vi "Path Array to Tree.vi"(7 "Path":path, 11 "Tree in":variant) -> (3 "Tree out":variant)   [LabVIEW 2023, in "VIDoc Printer.lvlib" / "VIDoc Printer.lvclass"]
uses:
  VIDoc Printer.lvclass
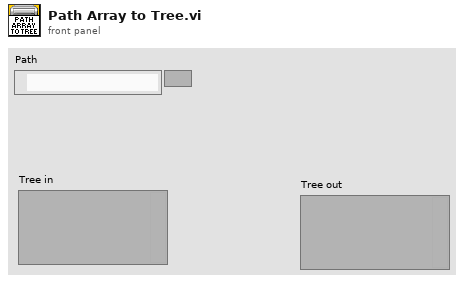
[diagram p1: front panel]
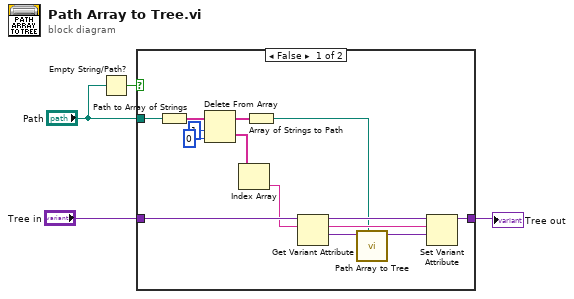
[diagram p0: block diagram]
diagram:
  n1 = Empty String/Path?(string/path="Path") -> (empty?=w2:bool)
  n2 = case shown="False" w2 {
    tunnel: [w16 w18] -> w4
    tunnel: "Tree in" -> [w13 w18]
    tunnel: "Path" -> [w12 _]
    frame False {
      n3 = Path to Array of Strings(0:w12) -> (2:w11:string[])  [unwired: 1 out]
      n4 = Delete From Array(array=w11, length=1, index=0) -> (deleted portion=w8:string[], array with subset deleted=w6:string[])
      n5 = Index Array(array=w8) -> (element=w7:string)  [unwired: 1 in]
      n6 = Array of Strings to Path(0:w6) -> (2:w5:path)  [unwired: 1 in]
      n7 = Get Variant Attribute(Variant=w13, name=w7) -> (duplicate Variant=w17:variant, value=w15:variant)  [unwired: 2 in, 2 out]
      n8 = call "Path Array to Tree.vi"("Path"=w5, "Tree in"=w15) -> ("Tree out"=w14:variant)  [unwired: 9 in]
      n9 = Set Variant Attribute(Variant=w17, name=w7, value=w14) -> (Variant out=w16:variant)  [unwired: 1 in, 2 out]
    }
    frame True {
    }
  }
  "Tree out" <- w4
